vi "IR - Stabilize.vi"(10 "IR Sensors":dbl[](array[numeric]), 11 "element":T1) -> (2 "appended array":dbl[](array[numeric]), 3 "logical AND":bool)   [LabVIEW 2019]
panel:
  out "Min":dbl
  out "Max":dbl
  out "0, 1":i16
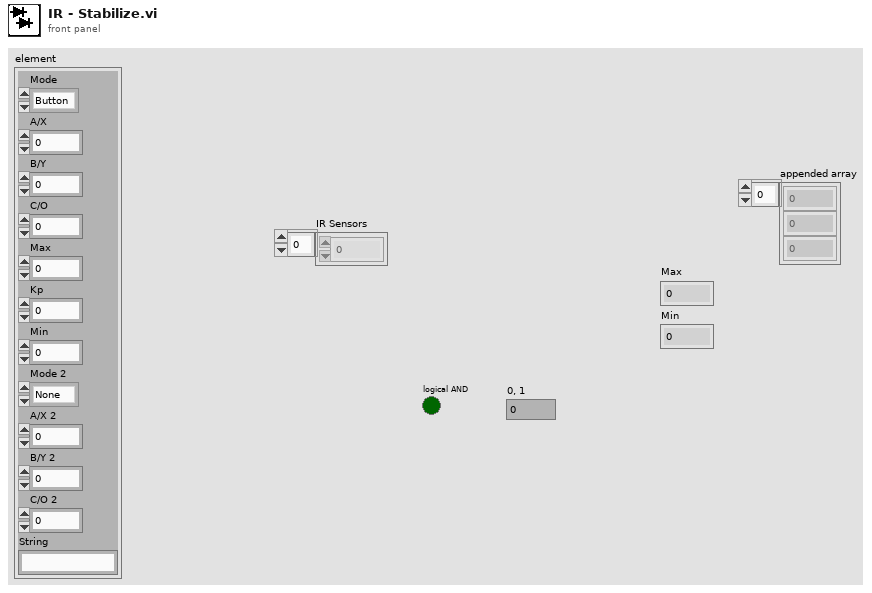
[diagram p1: front panel]
types:
  T1 = cluster{"Mode":enum16{"Button", "Encoder", "Delay", "IR Stop", "Line Stop"}, "A/X":dbl, "B/Y":dbl, "C/O":dbl, "Max":dbl, "Kp":dbl, "Min":dbl, "Mode 2":enum16{"None", "IR Stabilize", "Line Stabilize", "Encoder", "IR Stop", "Servo"}, "A/X 2":dbl, "B/Y 2":dbl, "C/O 2":dbl, "String":string}
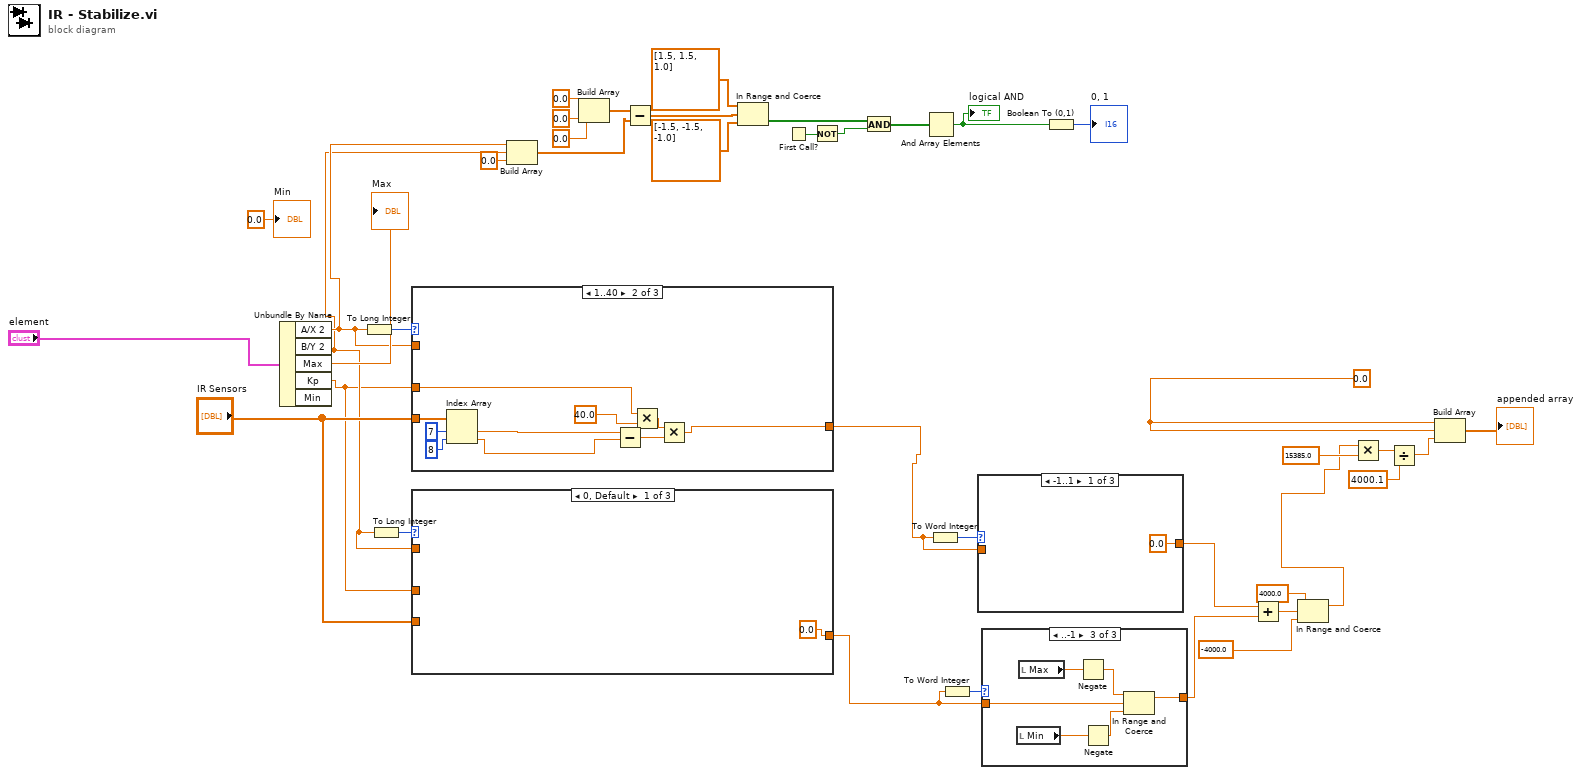
[diagram p0: block diagram]
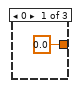
[diagram p2: hidden frame]
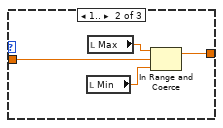
[diagram p3: hidden frame]
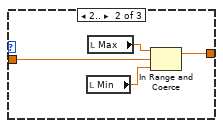
[diagram p4: hidden frame]
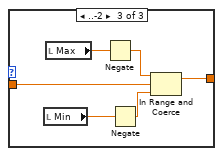
[diagram p5: hidden frame]
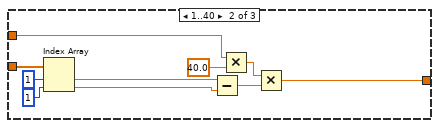
[diagram p6: hidden frame]
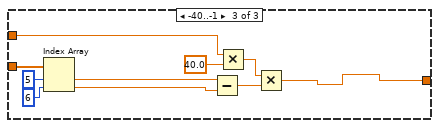
[diagram p7: hidden frame]
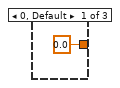
[diagram p8: hidden frame]
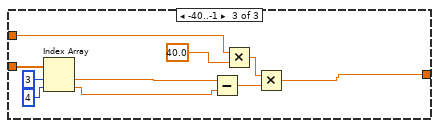
[diagram p9: hidden frame]
diagram:
  w20 = 0.0 ("element")
  n1 = Unbundle By Name("element") -> ("A/X 2"=w25:dbl, "B/Y 2"=w24:dbl, "Max"=→"Max":dbl, "Kp"=w12:dbl)  [unwired: 1 out]
  n2 = To Long Integer(number=w25) -> (32bit integer=w40:i32)
  n3 = To Long Integer(number=w24) -> (32bit integer=w39:i32)
  n4 = case shown="1..40" w40 {
    tunnel: "IR Sensors" -> [_ w51 w61]
    tunnel: w25 -> [_ _ _]
    tunnel: w12 -> [_ w46 w55]
    tunnel: [0.0 ("Max") w44 w54] -> w10
    frame 0, Default {
    }
    frame 1..40 {
      n5 = Index Array(array=w51, index #1=7 ("index"), index #2=8 ("index")) -> (element #1=w42:dbl, element #2=w43:dbl)
      n6 = Subtract(x=w42, y=w43) -> (x-y=w48:dbl)
      n7 = Multiply(x=w46, y=40.0) -> (x*y=w47:dbl)
      n8 = Multiply(x=w47, y=w48) -> (x*y=w44:dbl)
    }
    frame -40..-1 {
      n9 = Index Array(array=w61, index #1=3 ("index"), index #2=4 ("index")) -> (element #1=w53:dbl, element #2=w52:dbl)
      n10 = Subtract(x=w53, y=w52) -> (x-y=w58:dbl)
      n11 = Multiply(x=w55, y=40.0) -> (x*y=w56:dbl)
      n12 = Multiply(x=w56, y=w58) -> (x*y=w54:dbl)
    }
  }
  n13 = case shown="0, Default" w39 {
    tunnel: "IR Sensors" -> [_ w72 w82]
    tunnel: w24 -> [_ _ _]
    tunnel: w12 -> [_ w67 w77]
    tunnel: [0.0 ("Max") w66 w76] -> w8
    frame 0, Default {
    }
    frame 1..40 {
      n14 = Index Array(array=w72, index #1=1 ("index"), index #2=1 ("index")) -> (element #1=w65:dbl, element #2=w64:dbl)
      n15 = Subtract(x=w65, y=w64) -> (x-y=w69:dbl)
      n16 = Multiply(x=w67, y=40.0) -> (x*y=w68:dbl)
      n17 = Multiply(x=w68, y=w69) -> (x*y=w66:dbl)
    }
    frame -40..-1 {
      n18 = Index Array(array=w82, index #1=5 ("index"), index #2=6 ("index")) -> (element #1=w73:dbl, element #2=w74:dbl)
      n19 = Subtract(x=w73, y=w74) -> (x-y=w79:dbl)
      n20 = Multiply(x=w77, y=40.0) -> (x*y=w78:dbl)
      n21 = Multiply(x=w78, y=w79) -> (x*y=w76:dbl)
    }
  }
  n22 = Build Array(w25, w24, 0.0 ("element")) -> (w22:dbl[])
  n23 = Build Array(0.0 ("element"), 0.0 ("element"), 0.0 ("element")) -> (w26:dbl[])
  n24 = Subtract(x=w26, y=w22) -> (x-y=w21:dbl[])
  n25 = In Range and Coerce(upper limit=dbl[] [1.5, 1.5, 1.0], x=w21, lower limit=dbl[] [-1.5, -1.5, -1.0]) -> (In Range?=w35:bool[])  [unwired: 1 out]
  n26 = First Call?() -> (First Call?: T/F=w34:bool)
  n27 = Not(x=w34) -> (.not. x?=w33:bool)
  n28 = And(x=w35, y=w33) -> (x .and. y?=w32:bool[])
  n29 = And Array Elements(Boolean array=w32) -> (logical AND=w31:bool)
  "logical AND" <- w31
  n30 = To Word Integer(number=w10) -> (16bit integer=w13:i16)
  n31 = To Word Integer(number=w8) -> (16bit integer=w9:i16)
  n32 = case shown="-1..1" w13 {
    tunnel: [0.0 ("Max") w85 w92] -> w6
    tunnel: w10 -> [_ w84 w88]
    frame -1..1 {
    }
    frame 2.. {
      n33 = local read "Min"() -> (w86:dbl)
      n34 = local read "Max"() -> (w87:dbl)
      n35 = In Range and Coerce(upper limit=w87, x=w84, lower limit=w86) -> (coerced(x)=w85:dbl)  [unwired: 1 out]
    }
    frame ..-2 {
      n36 = local read "Min"() -> (w91:dbl)
      n37 = local read "Max"() -> (w93:dbl)
      n38 = Negate(x=w93) -> (-x=w89:dbl)
      n39 = Negate(x=w91) -> (-x=w90:dbl)
      n40 = In Range and Coerce(upper limit=w89, x=w88, lower limit=w90) -> (coerced(x)=w92:dbl)  [unwired: 1 out]
    }
  }
  n41 = case shown="..-1" w9 {
    tunnel: [0.0 ("Max") w96 w103] -> w7
    tunnel: w8 -> [_ w95 w99]
    frame 0 {
    }
    frame 1.. {
      n42 = local read "Min"() -> (w97:dbl)
      n43 = local read "Max"() -> (w98:dbl)
      n44 = In Range and Coerce(upper limit=w98, x=w95, lower limit=w97) -> (coerced(x)=w96:dbl)  [unwired: 1 out]
    }
    frame ..-1 {
      n45 = local read "Min"() -> (w102:dbl)
      n46 = local read "Max"() -> (w104:dbl)
      n47 = Negate(x=w104) -> (-x=w100:dbl)
      n48 = Negate(x=w102) -> (-x=w101:dbl)
      n49 = In Range and Coerce(upper limit=w100, x=w99, lower limit=w101) -> (coerced(x)=w103:dbl)  [unwired: 1 out]
    }
  }
  n50 = Boolean To (0,1)(Boolean=w31) -> (0, 1=→"0, 1":i16)
  n51 = Add(x=w6, y=w7) -> (x+y=w5:dbl)
  n52 = In Range and Coerce(upper limit=4000.0, x=w5, lower limit=-4000.0) -> (coerced(x)=w4:dbl)  [unwired: 1 out]
  n53 = Multiply(x=w4, y=15385.0) -> (x*y=w17:dbl)
  n54 = Divide(x=w17, y=4000.1) -> (x/y=w14:dbl)
  n55 = Build Array(w20, w20, w14) -> (→"appended array":dbl[])
  "Min" <- 0.0 ("Min")
